vi "List Glyphs.vi"(8 "error in (no error)":errorcluster, 11 "LV Awesome in":refnum<class "LV Awesome.lvclass">) -> (0 "error out":errorcluster, 2 "Glyphs":string[](array[string]), 3 "LV Awesome out":refnum<class "LV Awesome.lvclass">)   [LabVIEW 2020, in "LV-Awesome.lvlib" / "LV Awesome.lvclass"]
uses:
  LV Awesome.lvclass
  LV Awesome.lvclass/LV Awesome.ctl
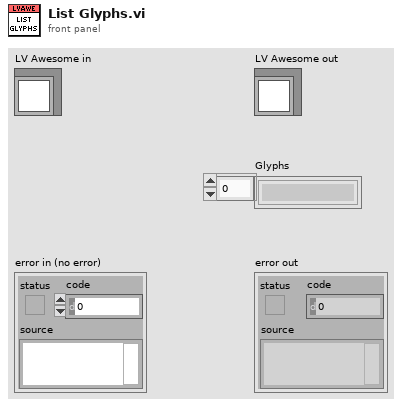
[diagram p1: front panel]
types:
  T1 = typedef "LV-Awesome.lvlib/LV Awesome.lvclass/Data.ctl" = cluster{"Glyphs":map{string, u32}, "Fonts":map{string, path}}
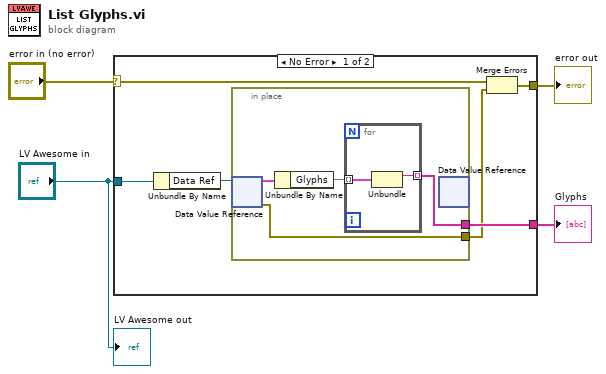
[diagram p0: block diagram]
diagram:
  n1 = case shown="No Error" "error in (no error)" {
    selector: "error in (no error)" -> [w7 w17]
    tunnel: "LV Awesome in" -> [w10 _]
    tunnel: [w8 _] -> w3
    tunnel: [w5 w17] -> w1
    frame No Error {
      n2 = Unbundle By Name(w10) -> ("Data Ref"=w9:refnum<data-value>)
      n3 = in-place {
        in-place-border: [w12] -> w8
        in-place-border: [w11] -> w6
        n4 = in-place-dvr #1(w9) -> (w14:T1, w11:errorcluster)
        n5 = Unbundle By Name(w14) -> ("Glyphs"=w13:map{string, u32})
        n6 = for {
          tunnel: w13 -> [w16] mode=indexing
          tunnel: [w15] -> w12 mode=indexing
          n7 = Unbundle(w16) -> ("Glyph"=w15:string)  [unwired: 1 out]
        }
        n8 = in-place-dvr #1() -> ()  [unwired: 1 in, 2 out]
      }
      n9 = Merge Errors(w7, w6) -> (w5:errorcluster)
    }
    frame Error {
    }
  }
  "error out" <- w1
  "Glyphs" <- w3
  "LV Awesome out" <- "LV Awesome in"
